vi "Write FoulVSS.vi"(8 "error in (no error)":errorcluster, 10 "FoulVSS":T1=enum."GOAL_KICK_ENEMY", 11 "Referee in":refnum<class "Referee.lvclass">) -> (0 "error out":errorcluster, 3 "Referee out":refnum<class "Referee.lvclass">)   [LabVIEW 2023, in "Referee.lvclass"]
uses:
  Referee.lvclass
  Command.ctl
  Referee.lvclass/Referee.ctl
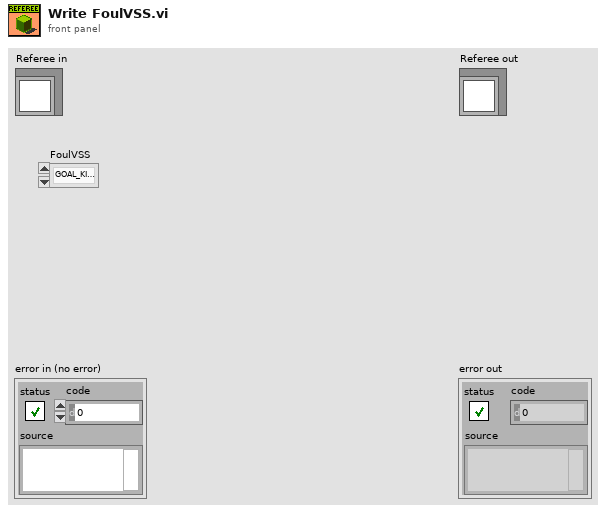
[diagram p1: front panel]
types:
  T1 = typedef "Command.ctl" = enum16{"AUTO", "GAME_ON", "STOP", "HALT", "KICKOFF_ALLY", "KICKOFF_ENEMY", "FREE_BALL", "GOAL_KICK_ENEMY", "GOAL_KICK_ALLY", "PENALTY_KICK_ENEMY", "PENALTY_KICK_ALLY", "FREE_KICK"}
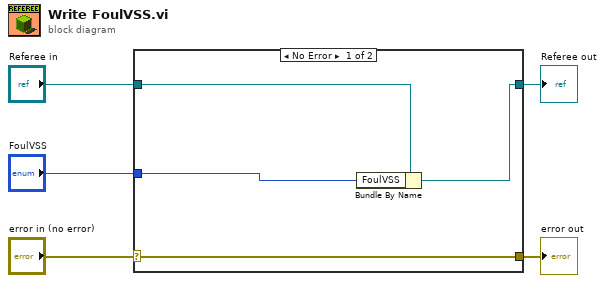
[diagram p0: block diagram]
diagram:
  n1 = case shown="No Error" "error in (no error)" {
    selector: "error in (no error)" -> [w9 w10]
    tunnel: [w9 w10] -> w4
    tunnel: [w7 w11] -> w2
    tunnel: "Referee in" -> [w8 w11]
    tunnel: "FoulVSS" -> [w6 _]
    frame No Error {
      n2 = Bundle By Name(cluster=w8, "FoulVSS"=w6) -> (w7:refnum<class "Referee.lvclass">)
    }
    frame Error {
    }
  }
  "error out" <- w4
  "Referee out" <- w2
